vi "9154 test.vi"() -> ()   [LabVIEW 2013]
uses:
  IP Source/Analog Replay/Settings.ctl
  IP Source/Analog Replay/Input.ctl
  IP Source/Analog Replay/Load Input.ctl
  IP Source/ECU Event/Timing/Measure Settings.ctl
  IP Source/ECU Event/Timing/Capture Output.ctl
  IP Source/APU/Settings.ctl
  IP Source/APU/Input.ctl
  IP Source/APU/Output.ctl
  IP Source/Version Token.ctl
  IP Source/ECU Event/Timing/Measure Output.ctl
  IP Source/APU/Shared Settings.ctl
  <vilib>/Platform/TimedLoop/XDataNode/timing_clust.ctl
  <vilib>/Platform/TimedLoop/XDataNode/nitl_modes.ctl
  <vilib>/Platform/TimedLoop/XDataNode/wakeup.ctl
  IP Source/ECU Event/Timing/Capture Settings.ctl
  <vilib>/rvi/DataTransferAndStorage/Container/Common/niFpgaContainerGetUniqueNameForEmu.vi
  <vilib>/rvi/DataTransferAndStorage/Container/Common/niFpgaContainerSetEmuInfo.vi
  <vilib>/rvi/eio/common/nirviEmuReportErrorAndStop.vi
  <vilib>/rvi/Emulation/niFpgaSctlEmulationGetInTimedLoop.vi
  <vilib>/rvi/Emulation/niFpgaEmulationReportErrorSimple.vi
  <vilib>/rvi/Emulation/niFpgaGetClockAttributes.vi
  <vilib>/rvi/Emulation/niFpgaCriticalErrorInLSC.vi
  <vilib>/rvi/eio/common/nirviEmuTemplateMethod_errors.vi
  <vilib>/Platform/TimedLoop/XDataNode/XDataNode.xnode
  <vilib>/rvi/LocalResourceManager/LocalResourceManager.xnode
  <vilib>/eio/EIONode/EIONode.xnode
  <vilib>/Platform/TimedLoop/XDataNode/XDNodeRunTimeDep.lvlib
  IP Source/Analog Replay/Analog Replay.lvlib
  IP Source/APU/APU.lvlib
  IP Source/ECU Event/Timing/ECU Event Timing.lvlib
  IP Source/Engine Simulation Toolkit.lvlib
panel:
  in  "shared settings.my apu":T1 {"cycle start" format="%#.15g"}
  out "measure output.fi 1":T2
  out "measure output.fi 2":T2
  out "measure output.fi 3":T2
  out "measure output.fi 4":T2
  out "measure output.fi 5":T2
  out "measure output.fi 6":T2
  out "measure output.fi 7":T2
  out "measure output.fi 8":T2
  out "measure output.fi 9":T2
  out "measure output.fi 10":T2
  out "measure output.spark 1":T2
  out "measure output.spark 2":T2
  out "measure output.spark 3":T2
  out "measure output.spark 4":T2
  out "measure output.spark 5":T2
  out "measure output.spark 6":T2
  out "measure output.spark 7":T2
  out "measure output.spark 8":T2
  out "measure output.spark 9":T2
  out "measure output.spark 10":T2
  in  "est.version":T3
  out "Output.my apu":T4 caption="output"
  in  "Input.my apu":T5 caption="input"
  in  "Settings.my apu":T6 caption="settings"
  out "Output.fi 7 shot":T7
  out "Output.fi 8 shot":T7
  out "Output.fi 9 shot":T7
  out "Output.fi 10 shot":T7
  in  "Settings.fi 7":T8
  in  "Settings.fi 8":T8
  in  "Settings.fi 9":T8
  in  "Settings.fi 10":T8
  out "Output.spark 7 shot 1":T7
  out "Output.spark 8 shot 1":T7
  out "Output.spark 9 shot 1":T7
  out "Output.spark 10 shot 1":T7
  in  "Settings.spark 7":T8
  in  "Settings.spark 8":T8
  in  "Settings.spark 9":T8
  in  "Settings.spark 10":T8
  out "Output.fi 1 shot 1":T7
  out "Output.fi 2 shot 1":T7
  out "Output.fi 3 shot 1":T7
  out "Output.fi 4 shot 1":T7
  out "Output.fi 5 shot 1":T7
  out "Output.fi 6 shot 1":T7
  in  "Settings.fi 1":T8
  in  "Settings.fi 2":T8
  in  "Settings.fi 3":T8
  in  "Settings.fi 4":T8
  in  "Settings.fi 5":T8
  in  "Settings.fi 6":T8
  out "Output.spark 1 shot 1":T7
  out "Output.spark 2 shot 1":T7
  out "Output.spark 3 shot 1":T7
  out "Output.spark 4 shot 1":T7
  out "Output.spark 5 shot 1":T7
  out "Output.spark 6 shot 1":T7
  in  "Settings.spark 1":T8
  in  "Settings.spark 2":T8
  in  "Settings.spark 3":T8
  in  "Settings.spark 4":T8
  in  "Settings.spark 5":T8
  in  "Settings.spark 6":T8
  in  "Input.replay 3":T9 caption="input"
  in  "Settings.replay 3":T10 caption="settings"
  in  "LoadInput.replay 3":T11={"Data"=[0, 0, 0, 0, 0, 0, 0, 0, 0, 0, 0, 0, 0, 0, 0, 0], "LoadOffset"=0, "Done"=FALSE} caption="input"
  in  "LoadInput.my replay":T11={"Data"=[0, 0, 0, 0, 0, 0, 0, 0, 0, 0, 0, 0, 0, 0, 0, 0], "LoadOffset"=0, "Done"=FALSE} caption="input"
  in  "LoadInput.my other replay":T11={"Data"=[0, 0, 0, 0, 0, 0, 0, 0, 0, 0, 0, 0, 0, 0, 0, 0], "LoadOffset"=0, "Done"=FALSE} caption="input"
  in  "Input.my replay":T9 caption="input"
  in  "Input.my other replay":T9 caption="input"
  in  "Settings.my other replay":T10 caption="settings"
  in  "Settings.my replay":T10 caption="settings"
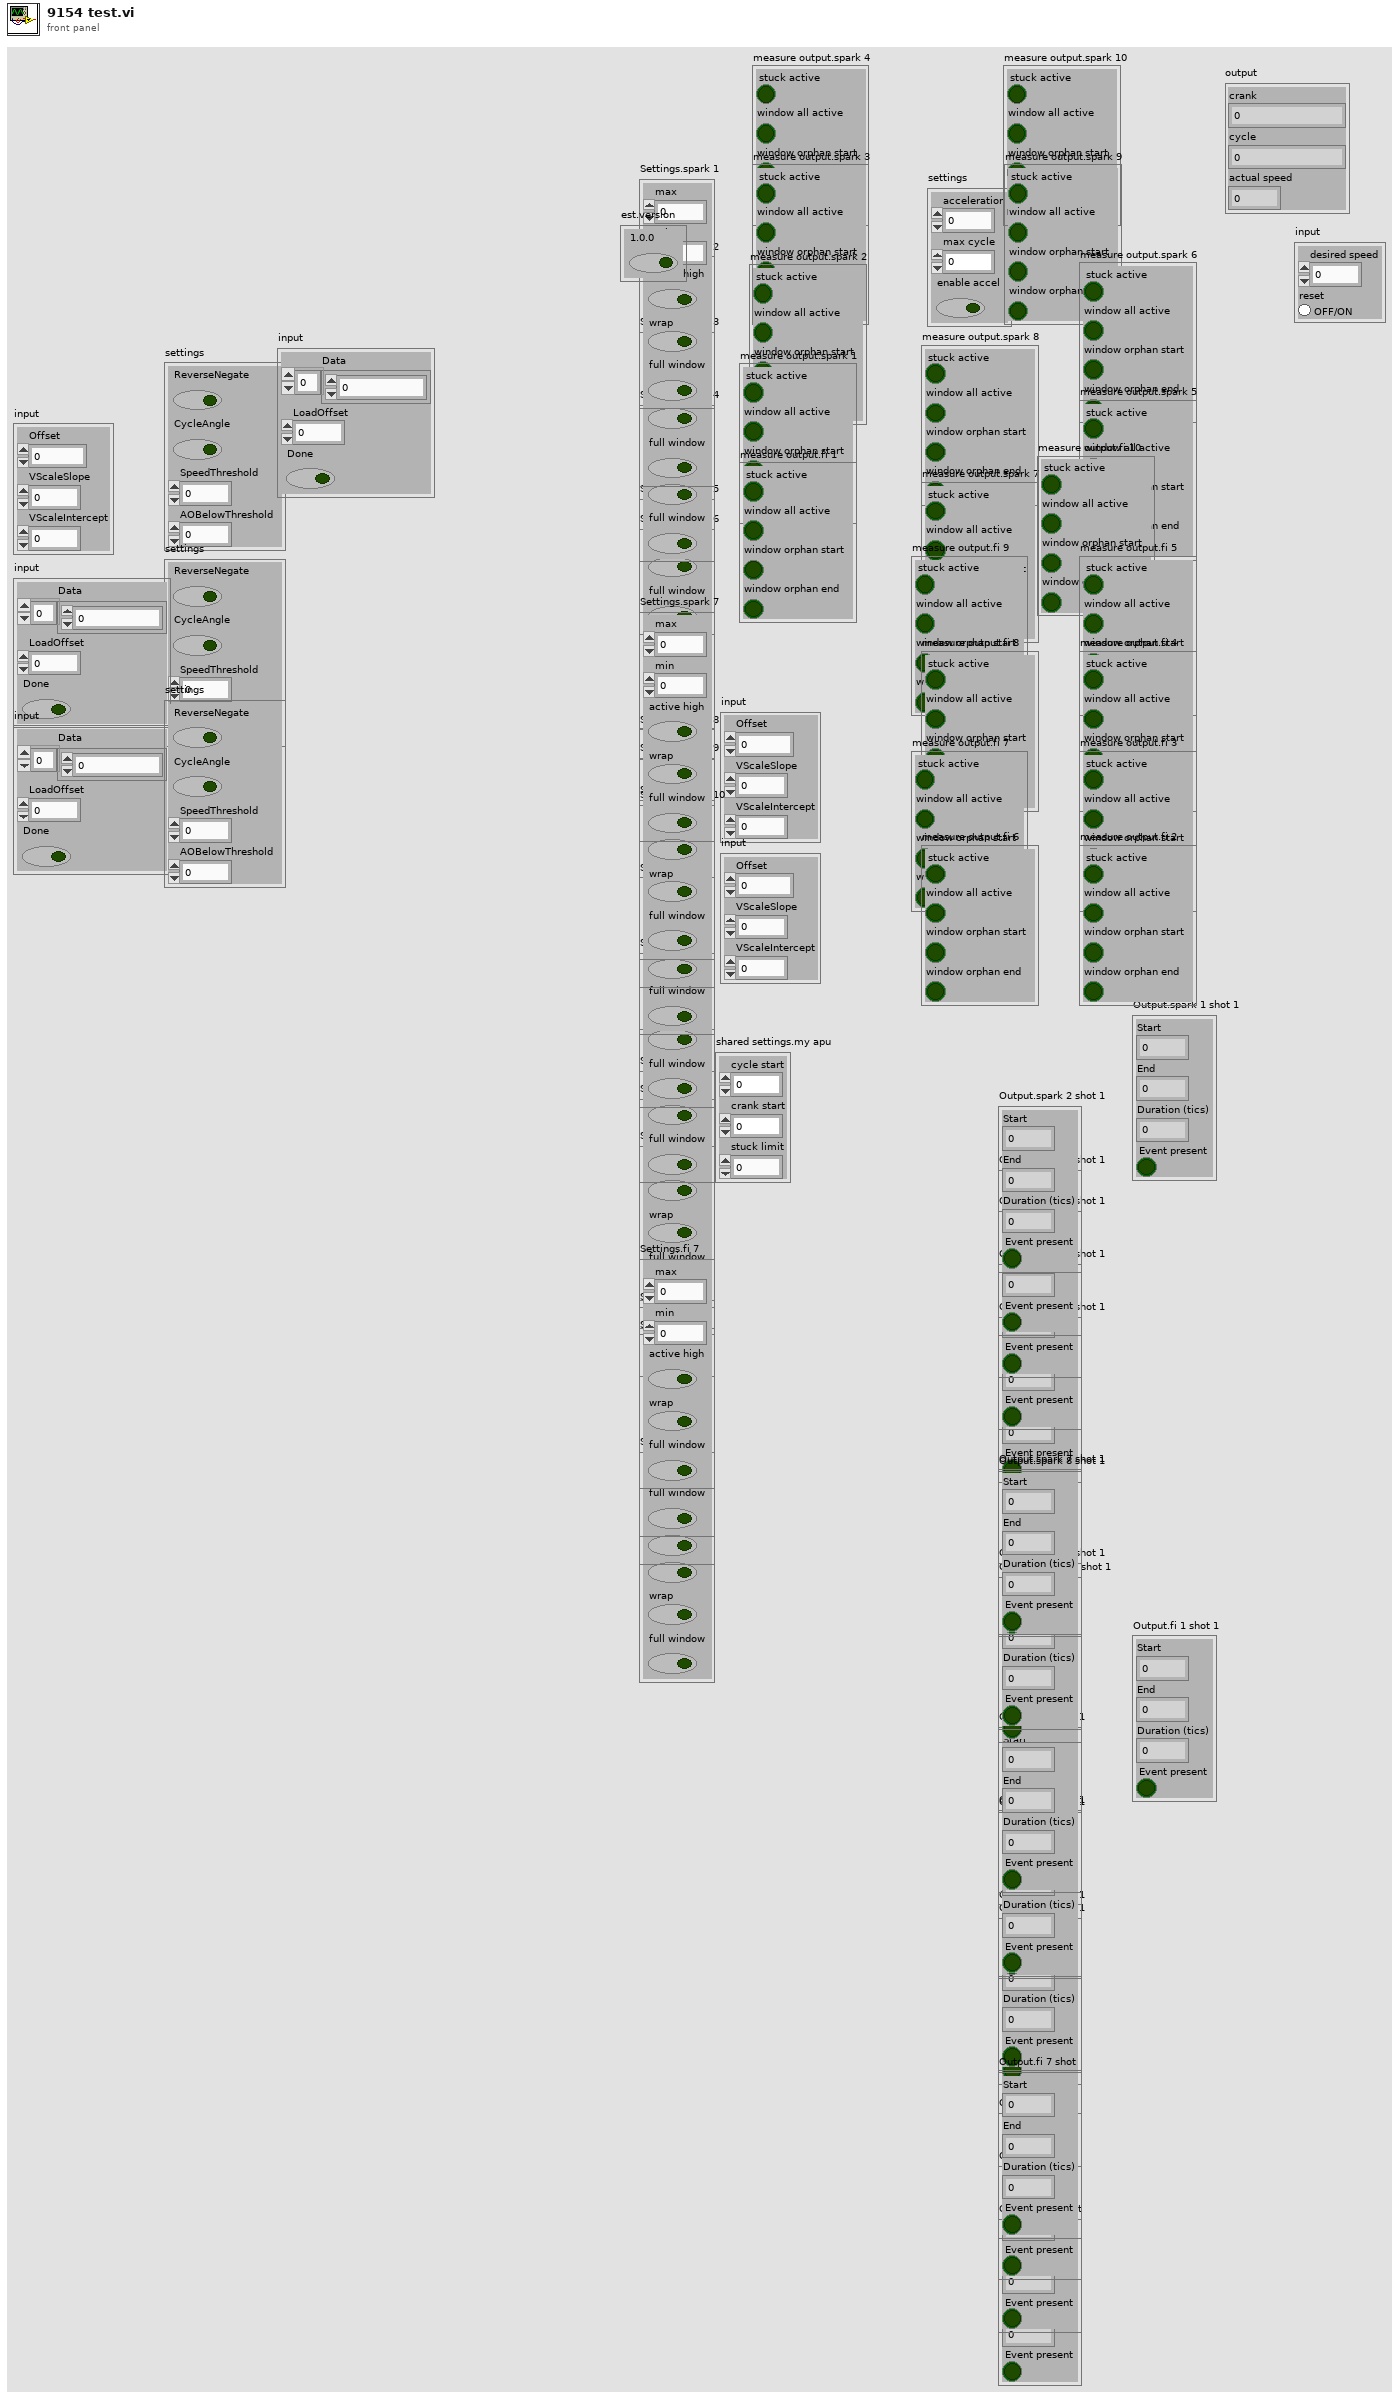
[diagram p1: front panel]
types:
  T1 = typedef "Engine Simulation Toolkit.lvlib/APU.lvlib/Shared Settings.ctl" = cluster{"cycle start":fxp<+,2,2>, "crank start":u16, "stuck limit":fxp<+,18,18>}
  T2 = typedef "Engine Simulation Toolkit.lvlib/ECU Event Timing.lvlib/Measure Output.ctl" = cluster{"stuck active":bool, "window all active":bool, "window orphan start":bool, "window orphan end":bool}
  T3 = typedef "Engine Simulation Toolkit.lvlib/Version Token.ctl" = cluster{"1.0.0":bool}
  T4 = typedef "Engine Simulation Toolkit.lvlib/APU.lvlib/Output.ctl" = cluster{"crank":u16, "cycle":u16, "actual speed":fxp<+/-,23,2>}
  T5 = typedef "Engine Simulation Toolkit.lvlib/APU.lvlib/Input.ctl" = cluster{"desired speed":fxp<+/-,23,2>, "reset":bool}
  T6 = typedef "Engine Simulation Toolkit.lvlib/APU.lvlib/Settings.ctl" = cluster{"acceleration":fxp<+,18,-20>, "max cycle":fxp<+,2,2>, "enable accel":bool}
  T7 = typedef "Engine Simulation Toolkit.lvlib/ECU Event Timing.lvlib/Capture Output.ctl" = cluster{"Start":u16, "End":u16, "Duration (tics)":fxp<+,18,18>, "Event present":bool}
  T8 = typedef "Engine Simulation Toolkit.lvlib/ECU Event Timing.lvlib/Measure Settings.ctl" = cluster{"max":u16, "min":u16, "active high":bool, "wrap":bool, "full window":bool}
  T9 = typedef "Engine Simulation Toolkit.lvlib/Analog Replay.lvlib/Input.ctl" = cluster{"Offset":i16, "VScaleSlope":fxp<+,18,6>, "VScaleIntercept":fxp<+/-,18,3>}
  T10 = typedef "Engine Simulation Toolkit.lvlib/Analog Replay.lvlib/Settings.ctl" = cluster{"ReverseNegate":bool, "CycleAngle":bool, "SpeedThreshold":fxp<+/-,23,2>, "AOBelowThreshold":i16}
  T11 = typedef "Engine Simulation Toolkit.lvlib/Analog Replay.lvlib/Load Input.ctl" = cluster{"Data":i16[], "LoadOffset":u16, "Done":bool}
  T12 = typedef "XDNodeRunTimeDep.lvlib/timing_clust.ctl" = cluster{"Expected End [f-1]":u64, "Actual End [f-1]":u64, "Finished Late? [f-1]":bool, "Expected End [i-1]":u64, "Actual End [i-1]":u64, "Finished Late? [i-1]":bool, "Expected Start [i]":u64, "Actual Start [i]":u64, "Expected Start [f]":u64, "Actual Start [f]":u64, "Source Name":string, "Structure Name":string, "Period":i64, "Deadline":i64, "Offset":i64, "Start":i64, "Priority":i32, "Timeout":i32, "Mode":T13, "Wakeup Reason":T14, "Error":errorcluster, "Source Type":string, "Secondary Source Type":string, "Global End Time":u64, "Global Start Time":u64, "Frame Duration":u64, "Iteration Duration":u64, "Assigned CPU":i32, "I/O Scan Engine Mode":u32}
  T13 = typedef "XDNodeRunTimeDep.lvlib/nitl_modes.ctl" = enum32{"No Change", "Process missed periods, maintain original phase", "Discard missed periods, maintain original phase", "Process missed periods, ignore original phase", "Discard missed periods, ignore original phase"}
  T14 = typedef "XDNodeRunTimeDep.lvlib/wakeup.ctl" = enum32{"Normal", "Aborted", "Asynchronous wakeup", "Timing source error", "Timed loop error", "Timeout"}
  T15 = typedef "Engine Simulation Toolkit.lvlib/APU.lvlib/Register Bus.ctl" = cluster{"Speed":refnum<k21>, "Crank Angle":refnum<k21>, "Cycle Angle":refnum<k21>, "Crank Count":refnum<k21>, "Cycle Count":refnum<k21>, "1.25 MHz Counter":refnum<k21>, "shared settings":T1}
  T16 = typedef "Engine Simulation Toolkit.lvlib/ECU Event Timing.lvlib/Capture Settings.ctl" = u8
  T17 = typedef "Engine Simulation Toolkit.lvlib/ECU Event Timing.lvlib/Measured Data.ctl" = cluster{"start":u16, "end":u16, "duration (tics)":fxp<+,18,18>, "window end":bool, "window begin":bool, "pulse end":bool, "pulse #":u8}
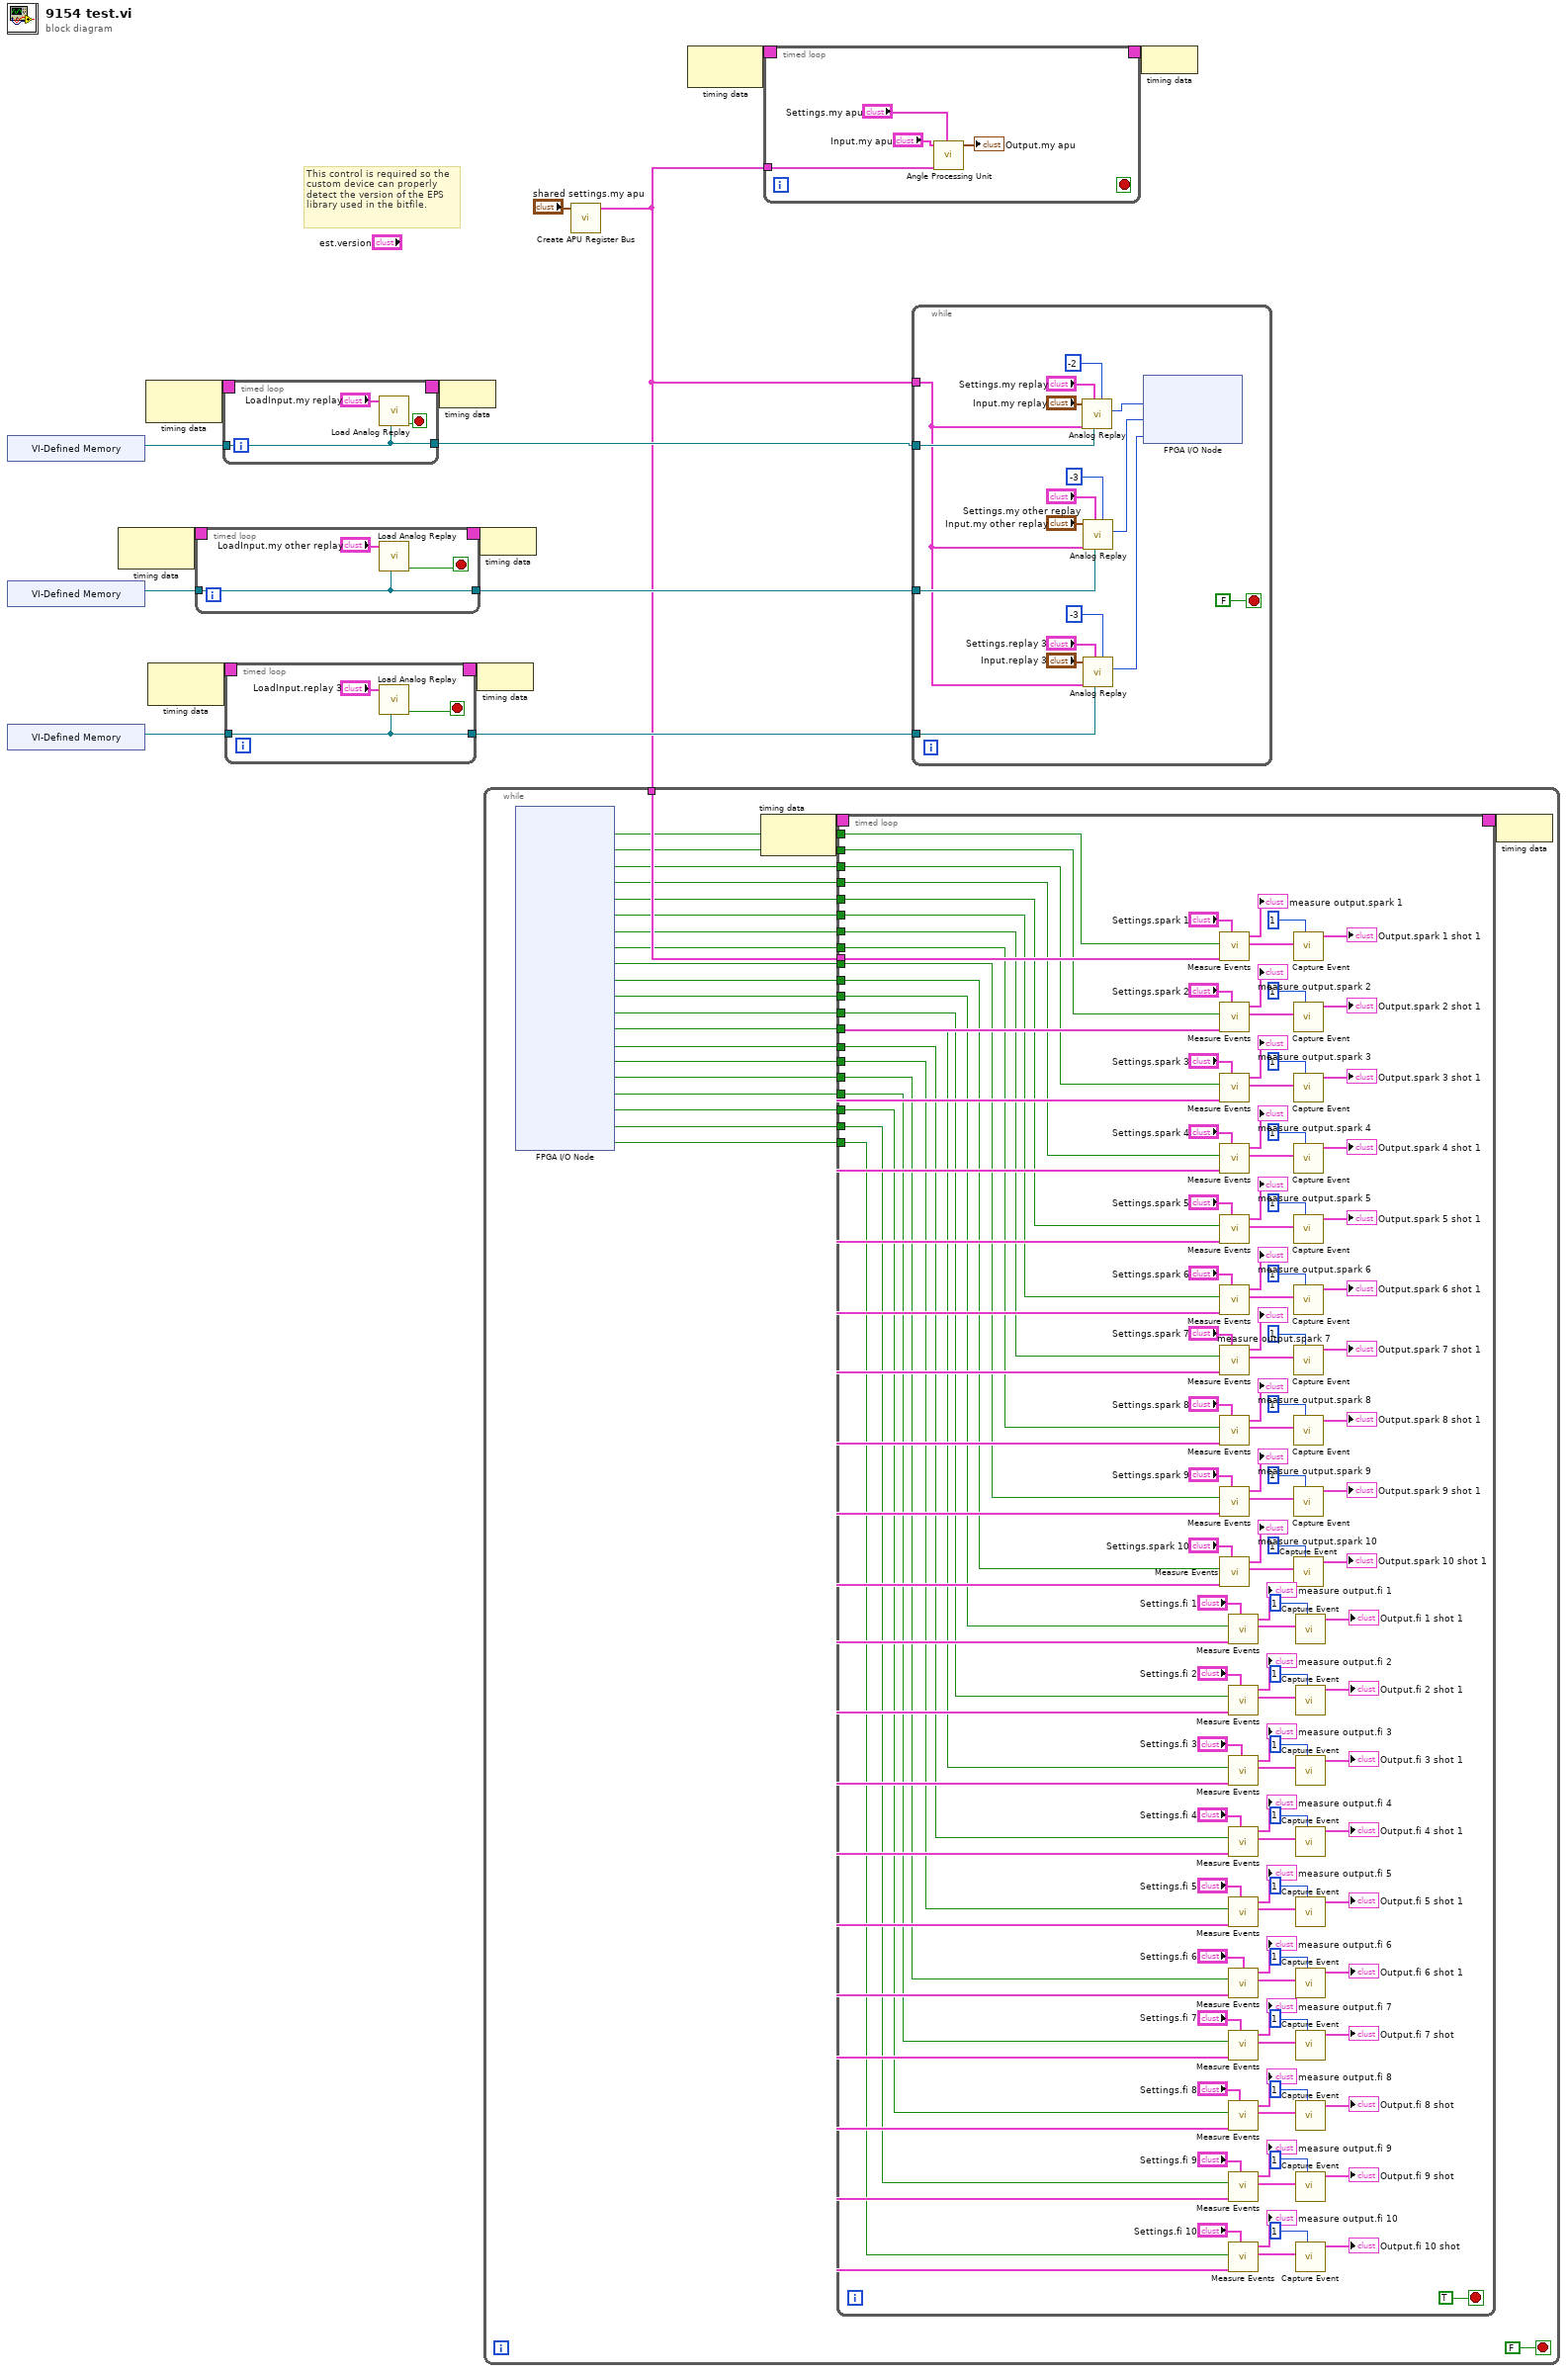
[diagram p0: block diagram]
diagram:
  # "This control is required so the custom device can properly detect the version of the EPS library used in the bitfile."
  n1 = xnode "VI-Defined Memory"() -> ("Memory Out"=w14:refnum<k21>)
  n2 = xnode "VI-Defined Memory"() -> ("Memory Out"=w15:refnum<k21>)
  n3 = xnode "VI-Defined Memory"() -> ("Memory Out"=w16:refnum<k21>)
  n4 = node-c288() -> (w10:T12)  [unwired: 1 in]
  n5 = node-c288() -> (w13:T12)  [unwired: 1 in]
  n6 = node-c288() -> (w7:T12)  [unwired: 1 in]
  n7 = timed-loop {
    timing: w10 -> [_]
    timing-out: [_] -> w9
    tunnel: w15 -> [w18]
    tunnel: [w18] -> w8
    stop <- w17 stop-if-true
    n8 = call "Load Analog Replay.vi"("memory"=w18, "load input.<user name>"="LoadInput.my other replay") -> ("done"=w17:bool)  [unwired: 9 in]
  }
  n9 = timed-loop {
    timing: w13 -> [_]
    timing-out: [_] -> w12
    tunnel: w14 -> [w22]
    tunnel: [w22] -> w11
    stop <- w23 stop-if-true
    n10 = call "Load Analog Replay.vi"("memory"=w22, "load input.<user name>"="LoadInput.my replay") -> ("done"=w23:bool)  [unwired: 9 in]
  }
  n11 = timed-loop {
    timing: w7 -> [_]
    timing-out: [_] -> w6
    tunnel: w16 -> [w27]
    tunnel: [w27] -> w5
    stop <- w28 stop-if-true
    n12 = call "Load Analog Replay.vi"("memory"=w27, "load input.<user name>"="LoadInput.replay 3") -> ("done"=w28:bool)  [unwired: 9 in]
  }
  n13 = node-c288(w12) -> ()
  n14 = node-c288(w6) -> ()
  n15 = node-c288(w9) -> ()
  n16 = call "Create APU Register Bus.vi"("shared settings.<user name>"="shared settings.my apu") -> ("register bus"=w2:T15)  [unwired: 10 in]
  n17 = while {
    tunnel: w2 -> [w53]
    stop <- FALSE stop-if-true
    n18 = xnode "FPGA I/O Node"() -> ("Mod2/DI0"=w52:bool, "Mod2/DI1"=w51:bool, "Mod2/DI2"=w50:bool, "Mod2/DI3"=w49:bool, "Mod2/DI4"=w48:bool, "Mod2/DI5"=w47:bool, "Mod2/DI6"=w46:bool, "Mod2/DI7"=w45:bool, "Mod2/DI8"=w44:bool, "Mod2/DI9"=w43:bool, "Mod2/DI10"=w42:bool, "Mod2/DI11"=w41:bool, "Mod2/DI12"=w40:bool, "Mod2/DI13"=w39:bool, "Mod2/DI14"=w38:bool, "Mod2/DI15"=w37:bool, "Mod2/DI16"=w36:bool, "Mod2/DI17"=w35:bool, "Mod2/DI18"=w34:bool, "Mod2/DI19"=w33:bool)  [unwired: 20 in, 20 out]
    n19 = node-c288() -> (w55:T12)  [unwired: 1 in]
    n20 = timed-loop {
      timing: w55 -> [_]
      timing-out: [_] -> w54
      tunnel: w53 -> [w177]
      tunnel: w52 -> [w155]
      tunnel: w51 -> [w154]
      tunnel: w50 -> [w153]
      tunnel: w49 -> [w152]
      tunnel: w48 -> [w151]
      tunnel: w47 -> [w150]
      tunnel: w46 -> [w149]
      tunnel: w45 -> [w148]
      tunnel: w44 -> [w147]
      tunnel: w43 -> [w146]
      tunnel: w42 -> [w145]
      tunnel: w41 -> [w144]
      tunnel: w40 -> [w143]
      tunnel: w39 -> [w142]
      tunnel: w38 -> [w141]
      tunnel: w37 -> [w140]
      tunnel: w36 -> [w139]
      tunnel: w35 -> [w138]
      tunnel: w34 -> [w137]
      tunnel: w33 -> [w136]
      stop <- TRUE stop-if-true
      n21 = call "Measure Events.vi"("settings.<user name>"="Settings.spark 1", "register bus"=w177, "event"=w155) -> ("measured data"=w97:T17, "status.<user name>"=→"measure output.spark 1":T2)  [unwired: 7 in]
      n22 = call "Measure Events.vi"("settings.<user name>"="Settings.spark 2", "register bus"=w177, "event"=w154) -> ("measured data"=w99:T17, "status.<user name>"=→"measure output.spark 2":T2)  [unwired: 7 in]
      n23 = call "Measure Events.vi"("settings.<user name>"="Settings.spark 3", "register bus"=w177, "event"=w153) -> ("measured data"=w101:T17, "status.<user name>"=→"measure output.spark 3":T2)  [unwired: 7 in]
      n24 = call "Measure Events.vi"("settings.<user name>"="Settings.spark 4", "register bus"=w177, "event"=w152) -> ("measured data"=w103:T17, "status.<user name>"=→"measure output.spark 4":T2)  [unwired: 7 in]
      n25 = call "Measure Events.vi"("settings.<user name>"="Settings.spark 5", "register bus"=w177, "event"=w151) -> ("measured data"=w105:T17, "status.<user name>"=→"measure output.spark 5":T2)  [unwired: 7 in]
      n26 = call "Measure Events.vi"("settings.<user name>"="Settings.spark 6", "register bus"=w177, "event"=w150) -> ("measured data"=w107:T17, "status.<user name>"=→"measure output.spark 6":T2)  [unwired: 7 in]
      n27 = call "Measure Events.vi"("settings.<user name>"="Settings.spark 7", "register bus"=w177, "event"=w149) -> ("measured data"=w109:T17, "status.<user name>"=→"measure output.spark 7":T2)  [unwired: 7 in]
      n28 = call "Measure Events.vi"("settings.<user name>"="Settings.spark 8", "register bus"=w177, "event"=w148) -> ("measured data"=w111:T17, "status.<user name>"=→"measure output.spark 8":T2)  [unwired: 7 in]
      n29 = call "Measure Events.vi"("settings.<user name>"="Settings.spark 9", "register bus"=w177, "event"=w147) -> ("measured data"=w113:T17, "status.<user name>"=→"measure output.spark 9":T2)  [unwired: 7 in]
      n30 = call "Measure Events.vi"("settings.<user name>"="Settings.spark 10", "register bus"=w177, "event"=w146) -> ("measured data"=w115:T17, "status.<user name>"=→"measure output.spark 10":T2)  [unwired: 7 in]
      n31 = call "Measure Events.vi"("settings.<user name>"="Settings.fi 1", "register bus"=w177, "event"=w145) -> ("measured data"=w117:T17, "status.<user name>"=→"measure output.fi 1":T2)  [unwired: 7 in]
      n32 = call "Measure Events.vi"("settings.<user name>"="Settings.fi 2", "register bus"=w177, "event"=w144) -> ("measured data"=w119:T17, "status.<user name>"=→"measure output.fi 2":T2)  [unwired: 7 in]
      n33 = call "Measure Events.vi"("settings.<user name>"="Settings.fi 3", "register bus"=w177, "event"=w143) -> ("measured data"=w121:T17, "status.<user name>"=→"measure output.fi 3":T2)  [unwired: 7 in]
      n34 = call "Measure Events.vi"("settings.<user name>"="Settings.fi 4", "register bus"=w177, "event"=w142) -> ("measured data"=w123:T17, "status.<user name>"=→"measure output.fi 4":T2)  [unwired: 7 in]
      n35 = call "Measure Events.vi"("settings.<user name>"="Settings.fi 5", "register bus"=w177, "event"=w141) -> ("measured data"=w125:T17, "status.<user name>"=→"measure output.fi 5":T2)  [unwired: 7 in]
      n36 = call "Measure Events.vi"("settings.<user name>"="Settings.fi 6", "register bus"=w177, "event"=w140) -> ("measured data"=w127:T17, "status.<user name>"=→"measure output.fi 6":T2)  [unwired: 7 in]
      n37 = call "Measure Events.vi"("settings.<user name>"="Settings.fi 7", "register bus"=w177, "event"=w139) -> ("measured data"=w129:T17, "status.<user name>"=→"measure output.fi 7":T2)  [unwired: 7 in]
      n38 = call "Measure Events.vi"("settings.<user name>"="Settings.fi 8", "register bus"=w177, "event"=w138) -> ("measured data"=w131:T17, "status.<user name>"=→"measure output.fi 8":T2)  [unwired: 7 in]
      n39 = call "Measure Events.vi"("settings.<user name>"="Settings.fi 9", "register bus"=w177, "event"=w137) -> ("measured data"=w134:T17, "status.<user name>"=→"measure output.fi 9":T2)  [unwired: 7 in]
      n40 = call "Measure Events.vi"("settings.<user name>"="Settings.fi 10", "register bus"=w177, "event"=w136) -> ("measured data"=w135:T17, "status.<user name>"=→"measure output.fi 10":T2)  [unwired: 7 in]
      n41 = call "Capture Event.vi"("event # to capture"=T16 1 ("Settings.spark 1 shot 1"), "measured data"=w97) -> ("capture.<user name>"=→"Output.spark 1 shot 1":T7)  [unwired: 9 in]
      n42 = call "Capture Event.vi"("event # to capture"=T16 1 ("Settings.spark 2 shot 1"), "measured data"=w99) -> ("capture.<user name>"=→"Output.spark 2 shot 1":T7)  [unwired: 9 in]
      n43 = call "Capture Event.vi"("event # to capture"=T16 1 ("Settings.spark 3 shot 1"), "measured data"=w101) -> ("capture.<user name>"=→"Output.spark 3 shot 1":T7)  [unwired: 9 in]
      n44 = call "Capture Event.vi"("event # to capture"=T16 1 ("Settings.spark 4 shot 1"), "measured data"=w103) -> ("capture.<user name>"=→"Output.spark 4 shot 1":T7)  [unwired: 9 in]
      n45 = call "Capture Event.vi"("event # to capture"=T16 1 ("Settings.spark 5 shot 1"), "measured data"=w105) -> ("capture.<user name>"=→"Output.spark 5 shot 1":T7)  [unwired: 9 in]
      n46 = call "Capture Event.vi"("event # to capture"=T16 1 ("Settings.spark 6 shot 1"), "measured data"=w107) -> ("capture.<user name>"=→"Output.spark 6 shot 1":T7)  [unwired: 9 in]
      n47 = call "Capture Event.vi"("event # to capture"=T16 1 ("Settings.spark 3 shot 1"), "measured data"=w109) -> ("capture.<user name>"=→"Output.spark 7 shot 1":T7)  [unwired: 9 in]
      n48 = call "Capture Event.vi"("event # to capture"=T16 1 ("Settings.spark 4 shot 1"), "measured data"=w111) -> ("capture.<user name>"=→"Output.spark 8 shot 1":T7)  [unwired: 9 in]
      n49 = call "Capture Event.vi"("event # to capture"=T16 1 ("Settings.spark 5 shot 1"), "measured data"=w113) -> ("capture.<user name>"=→"Output.spark 9 shot 1":T7)  [unwired: 9 in]
      n50 = call "Capture Event.vi"("event # to capture"=T16 1 ("Settings.spark 6 shot 1"), "measured data"=w115) -> ("capture.<user name>"=→"Output.spark 10 shot 1":T7)  [unwired: 9 in]
      n51 = call "Capture Event.vi"("event # to capture"=T16 1 ("Settings.fi 1 shot 1"), "measured data"=w117) -> ("capture.<user name>"=→"Output.fi 1 shot 1":T7)  [unwired: 9 in]
      n52 = call "Capture Event.vi"("event # to capture"=T16 1 ("Settings.fi 2 shot 1"), "measured data"=w119) -> ("capture.<user name>"=→"Output.fi 2 shot 1":T7)  [unwired: 9 in]
      n53 = call "Capture Event.vi"("event # to capture"=T16 1 ("Settings.fi 3 shot 1"), "measured data"=w121) -> ("capture.<user name>"=→"Output.fi 3 shot 1":T7)  [unwired: 9 in]
      n54 = call "Capture Event.vi"("event # to capture"=T16 1 ("Settings.fi 4 shot 1"), "measured data"=w123) -> ("capture.<user name>"=→"Output.fi 4 shot 1":T7)  [unwired: 9 in]
      n55 = call "Capture Event.vi"("event # to capture"=T16 1 ("Settings.fi 5 shot 1"), "measured data"=w125) -> ("capture.<user name>"=→"Output.fi 5 shot 1":T7)  [unwired: 9 in]
      n56 = call "Capture Event.vi"("event # to capture"=T16 1 ("Settings.fi 6 shot 1"), "measured data"=w127) -> ("capture.<user name>"=→"Output.fi 6 shot 1":T7)  [unwired: 9 in]
      n57 = call "Capture Event.vi"("event # to capture"=T16 1 ("Settings.fi 3 shot 1"), "measured data"=w129) -> ("capture.<user name>"=→"Output.fi 7 shot":T7)  [unwired: 9 in]
      n58 = call "Capture Event.vi"("event # to capture"=T16 1 ("Settings.fi 4 shot 1"), "measured data"=w131) -> ("capture.<user name>"=→"Output.fi 8 shot":T7)  [unwired: 9 in]
      n59 = call "Capture Event.vi"("event # to capture"=T16 1 ("Settings.fi 5 shot 1"), "measured data"=w134) -> ("capture.<user name>"=→"Output.fi 9 shot":T7)  [unwired: 9 in]
      n60 = call "Capture Event.vi"("event # to capture"=T16 1 ("Settings.fi 6 shot 1"), "measured data"=w135) -> ("capture.<user name>"=→"Output.fi 10 shot":T7)  [unwired: 9 in]
    }
    n61 = node-c288(w54) -> ()
  }
  n62 = node-c288() -> (w4:T12)  [unwired: 1 in]
  n63 = timed-loop {
    timing: w4 -> [_]
    timing-out: [_] -> w3
    tunnel: w2 -> [w182]
    stop <- _ stop-if-true
    n64 = call "Angle Processing Unit.vi"("settings.<user name>"="Settings.my apu", "register bus"=w182, "input.<user name>"="Input.my apu") -> ("output.<user name>"=→"Output.my apu":T4)  [unwired: 8 in]
  }
  n65 = while {
    tunnel: w11 -> [w204]
    tunnel: w2 -> [w188]
    tunnel: w8 -> [w201]
    tunnel: w5 -> [w198]
    stop <- FALSE stop-if-true
    n66 = call "Analog Replay.vi"("shift"=i8 -2, "memory"=w204, "settings.<user name>"="Settings.my replay", "register bus"=w188, "input.<user name>"="Input.my replay") -> ("analog value"=w191:i16)  [unwired: 6 in]
    n67 = call "Analog Replay.vi"("shift"=i8 -3, "memory"=w201, "settings.<user name>"="Settings.my other replay", "register bus"=w188, "input.<user name>"="Input.my other replay") -> ("analog value"=w190:i16)  [unwired: 6 in]
    n68 = call "Analog Replay.vi"("shift"=i8 -3, "memory"=w198, "settings.<user name>"="Settings.replay 3", "register bus"=w188, "input.<user name>"="Input.replay 3") -> ("analog value"=w189:i16)  [unwired: 6 in]
    n69 = xnode "FPGA I/O Node"("Mod1/AO0"=w191, "Mod1/AO1"=w190, "Mod1/AO2"=w189) -> ()  [unwired: 3 in, 3 out]
  }
  n70 = node-c288(w3) -> ()
